vi "qPMI.vi"(0 "System no.":i32=1 min=1 max=4 step=1, 2 "Axes to query":string[](array[string]), 3 "All axes?":bool, 4 "Axis identifier?":bool=TRUE, 5 "error in":errorcluster) -> (14 "Negative limit?":dbl[](array[numeric]) format="%.6f", 19 "error out":errorcluster)   [LabVIEW 2026]
doc: "Returns minimum position limit of queried axes. Old command-please use NLM? if the system supports that command.\n\nE-516: If All axes = TRUE, then Axis identifier must be TRUE"
panel:
  # "Returns minimum position limit of queried axes. (new: NLM?)"
  # "If all axes: use"
  # "Query"
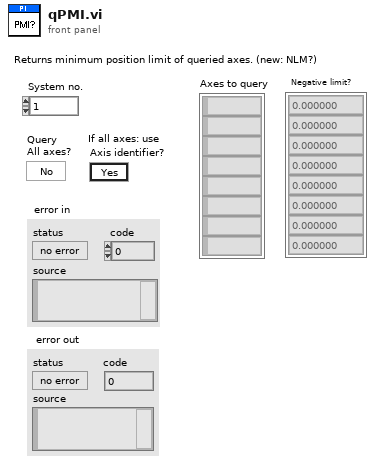
[diagram p1: front panel]
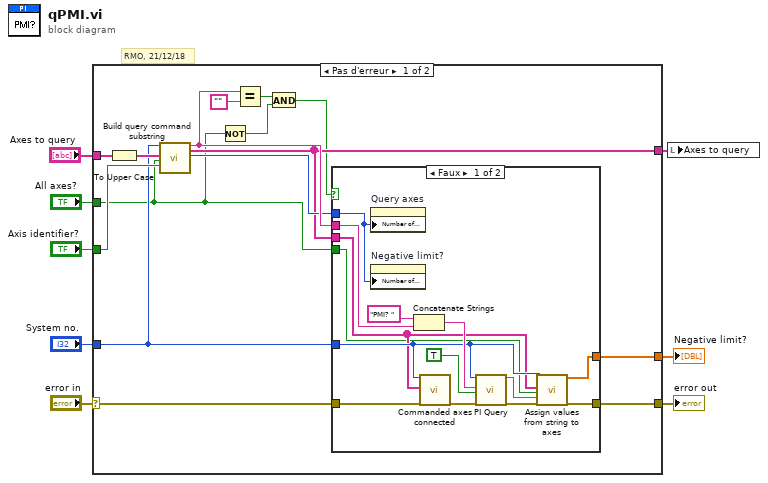
[diagram p0: block diagram]
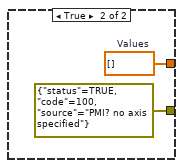
[diagram p2: hidden frame]
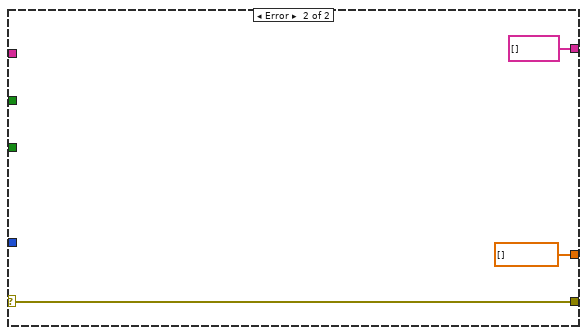
[diagram p3: hidden frame]
diagram:
  # "RMO, 21/12/18"
  n1 = case shown="Pas d'erreur" "error in" {
    selector: "error in" -> [w11 w40]
    tunnel: [w23 dbl[] [] ("Values")] -> w8
    tunnel: "Axes to query" -> [w22 _]
    tunnel: [w10 w40] -> w6
    tunnel: "Axis identifier?" -> [w19 _]
    tunnel: "System no." -> [w16 _]
    tunnel: [w15 string[] [] ("Axes to query out")] -> w3
    tunnel: "All axes?" -> [w14 _]
    frame No Error {
      n2 = To Upper Case(1:w22) -> (0:w20:string[])
      n3 = call "Build query command substring.vi"("System no."=w16, "Axes to query in"=w20, "Query\nAll axes?"=w14, "For all axes: use\nAxis identifier?"=w19) -> ("Command substring"=w18:string, "Axes to query out"=w15:string[], "Number of rows"=w17:u32)  [unwired: 2 in, 11 out]
      n4 = Not(x=w14) -> (.not. x?=w12:bool)
      n5 = Equal?(x=w18, y="" ("x")) -> (x = y?=w13:bool)
      n6 = And(x=w13, y=w12) -> (x .and. y?=w9:bool)
      n7 = case shown="Faux" w9 {
        tunnel: [w34 w38] -> w23
        tunnel: w18 -> [w33 _]
        tunnel: w17 -> [w32 _]
        tunnel: w16 -> [w31 _]
        tunnel: w15 -> [w30 _]
        tunnel: w14 -> [w29 _]
        tunnel: w11 -> [w27 _]
        tunnel: [w26 errorcluster {"status"=TRUE, "code"=100, "source"="PMI? no axis specified"} ("error out")] -> w10
        frame False {
          n8 = property on="Query axes" class="Tabl (strict)"("Number of Rows"=w32) -> ()  [unwired: 2 in, 2 out]
          n9 = property on="Negative limit?" class="Tabl (strict)"("Number of Rows"=w32) -> ()  [unwired: 2 in, 2 out]
          n10 = Concatenate Strings("PMI? ", w33) -> (w35:string)
          n11 = call "Commanded axes connected.vi"("System no."=w31, "Commanded axes"=w30, "error in"=w27) -> ("error out"=w28:errorcluster)  [unwired: 1 in, 15 out]
          n12 = call "PI Query.vi"("System no."=w31, "String to send"=w35, "Attach termination char.?"=TRUE ("Attach Linefeed?"), "error in"=w28) -> ("String read"=w24:string, "error out"=w25:errorcluster)  [unwired: 3 in, 11 out]
          n13 = call "Assign values from string to axes.vi"("System no."=w31, "Queried axes"=w30, "All axes queried?"=w29, "Input String"=w24, "error in"=w25) -> ("Values"=w34:dbl[], "error out"=w26:errorcluster)  [unwired: 4 in, 9 out]
        }
        frame True {
          w38 = dbl[] []  # Values
        }
      }
    }
    frame Error {
    }
  }
  "error out" <- w6
  "Negative limit?" <- w8
  n14 = local write "Axes to query"(w3) -> ()
